vi "utf-8 - text.vi"   [LabVIEW 2021]
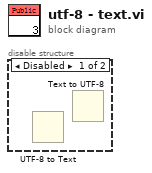
[diagram p0: block diagram]
diagram:
  n1 = disable-structure shown="Disabled" {
    frame Disabled {
      n2 = UTF-8 to Text() -> ()  [unwired: 3 in, 2 out]
      n3 = Text to UTF-8() -> ()  [unwired: 3 in, 2 out]
    }
    frame Enabled {
    }
  }
